vi "Durchfluss aendern bei Analysatorstatus.vi"(6 "Aktion":T1, 8 "error in (no error)":errorcluster caption="Fehler (Eingang, kein Fehler)", 11 "Status Analysatoren":T2) -> (0 "error out":errorcluster caption="Fehler (Ausgang)", 3 "Durchflussänderung":bool)   [LabVIEW 2020, in "Anlagengrenzwerte.lvlib"]
uses:
  Anlagengrenzwerte.lvlib
  Status Analysatoren/Status.ctl
  Aktion Durchflussaenderung.ctl
  FGV Anlagengrenzwerte Aktionen.ctl
  Status Analysatoren/Status Analysatoren.lvlib
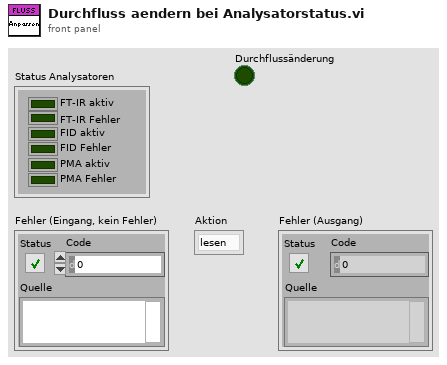
[diagram p1: front panel]
types:
  T1 = typedef "Anlagengrenzwerte.lvlib/Aktion Durchflussaenderung.ctl" = enum16{"lesen", "Statusänderung", "Reset"}
  T2 = typedef "Status Analysatoren.lvlib/Status.ctl" = cluster{"FT-IR aktiv":bool, "FT-IR Fehler":bool, "FID aktiv":bool, "FID Fehler":bool, "PMA aktiv":bool, "PMA Fehler":bool}
  T3 = typedef "Anlagengrenzwerte.lvlib/FGV Anlagengrenzwerte Aktionen.ctl" = enum16{"Lesen", "Grenzwerte schreiben"}
  T4 = typedef "Anlagengrenzwerte.lvlib/Anlagen-Grenzwerte Anzeige.ctl" = cluster{"Eingangsdruck FT-IR:":T5, "Durchfluss FT-IR:":T5, "Durchfluss CalGas:":T5, "Druck Ausgang:":T5, "Druck Kalter Block:":T5, "Heizleitungen intern:":T5, "Heizleitung zu FT-IR:":T5, "Heizung Filterblock:":T5, "Heizung Pumpe:":T5, "Heizleitung Extern SP1:":T5, "Heizleitung Extern SP2:":T5, "FT-IR Heizung Messzelle:":T5, "Schaltschranktemperatur:":T5, "Gaskühler:":T5}
  T5 = typedef "Anlagengrenzwerte.lvlib/Anlagen-Parameter Anzeige.ctl" = cluster{"Sollwert":sgl, "Warn-Min":sgl, "Warn-Max":sgl, "Abschalt-Min":sgl, "Abschalt-Max":sgl, "Regler":u16}
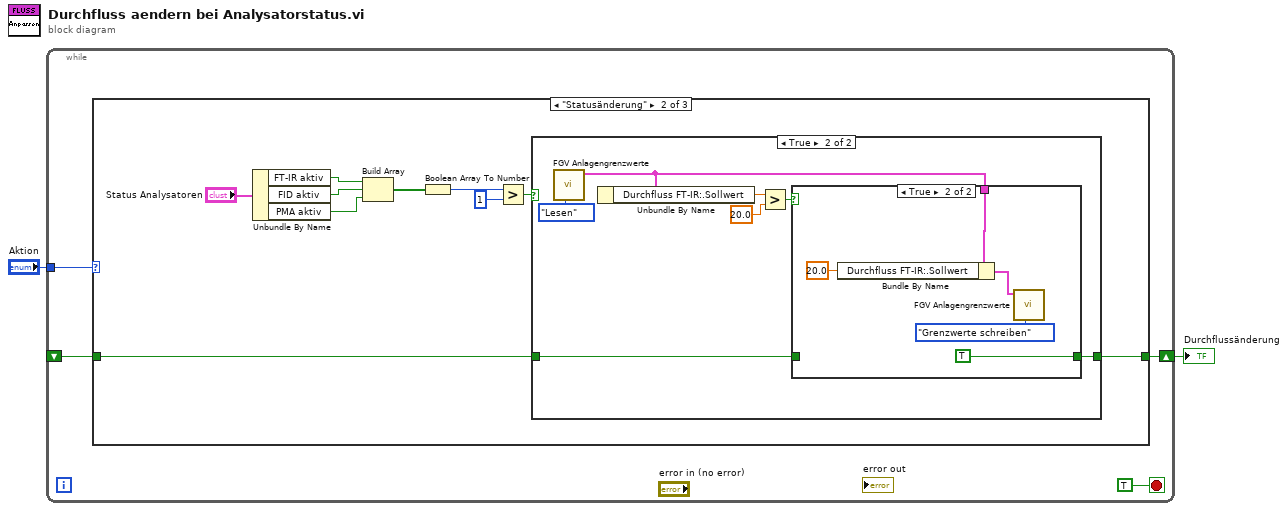
[diagram p0: block diagram]
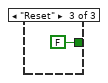
[diagram p5: hidden frame]
diagram:
  n1 = while {
    shift-right: [w5] -> w1
    shift-left: _ -> [w4]
    tunnel: "Aktion" -> [w3]
    stop <- TRUE stop-if-true
    n2 = case shown="\"Statusänderung\"" w3 {
      tunnel: [w7 w9 FALSE] -> w5
      tunnel: w4 -> [w7 w8 _]
      frame "lesen", Default {
      }
      frame "Statusänderung" {
        n3 = Unbundle By Name("Status Analysatoren") -> ("FT-IR aktiv"=w16:bool, "FID aktiv"=w15:bool, "PMA aktiv"=w14:bool)
        n4 = Build Array(w16, w15, w14) -> (w13:bool[])
        n5 = Boolean Array To Number(Boolean array=w13) -> (number=w12:u32)
        n6 = Greater?(x=w12, y=u32 1) -> (0:w10:bool)
        n7 = case shown="True" w10 {
          tunnel: [w18 w20] -> w9
          tunnel: w8 -> [w18 w19]
          frame False {
          }
          frame True {
            n8 = call "FGV Anlagengrenzwerte.vi"("Aktion"=FGV_Anlagengrenzwerte_Aktionen."Lesen") -> ("Anlagen-Grenzwerte Anzeige"=w24:T4)  [unwired: 10 in]
            n9 = Unbundle By Name(w24) -> ("Durchfluss FT-IR:.Sollwert"=w23:sgl)
            n10 = Greater?(x=w23, y=sgl 20.0) -> (0:w21:bool)
            n11 = case shown="True" w21 {
              tunnel: w24 -> [_ w29]
              tunnel: [w26 TRUE] -> w20
              tunnel: w19 -> [w26 _]
              frame False {
              }
              frame True {
                n12 = Bundle By Name(cluster=w29, "Durchfluss FT-IR:.Sollwert"=sgl 20.0) -> (w30:T4)
                n13 = call "FGV Anlagengrenzwerte.vi"("Aktion"=FGV_Anlagengrenzwerte_Aktionen."Grenzwerte schreiben", "Anlagen-Grenzwerte Anzeige"=w30) -> ()  [unwired: 9 in, 1 out]
              }
            }
          }
        }
      }
      frame "Reset" {
      }
    }
  }
  "Durchflussänderung" <- w1
